vi "peak - geometry fit.vi"(10 "omega":dbl[](array[numeric]), 11 "linear z":cdb[](array[numeric])) -> (0 "gamma":dbl, 1 "omega":dbl)   [LabVIEW 2015]
uses:
  <vilib>/Analysis/6fits.llb/Curve Fitting Criteria.ctl
  <vilib>/Analysis/NI_AALPro.lvlib
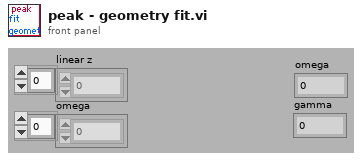
[diagram p1: front panel]
types:
  T1 = typedef "NI_AALPro.lvlib/Curve Fitting Criteria.ctl" = u16
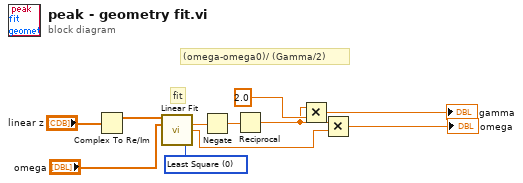
[diagram p0: block diagram]
diagram:
  w11 = T1 0 items=["Least Square", "Least Absolute Residual", "Bisquare"] ("method")
  # "(omega-omega0)/ (Gamma/2)"
  # "fit"
  n1 = Complex To Re/Im(x + iy="linear z") -> (x=w2:dbl[])  [unwired: 1 out]
  n2 = call <vilib>:"Linear Fit.vi"("Y"=w2, "X"="omega", "method"=w11) -> ("slope"=w9:dbl, "intercept"=w7:dbl)  [unwired: 8 in, 3 out]
  n3 = Negate(x=w9) -> (-x=w8:dbl)
  n4 = Reciprocal(x=w8) -> (1/x=w6:dbl)
  n5 = Multiply(x=w6, y=2.0) -> (x*y=→"gamma":dbl)
  n6 = Multiply(x=w6, y=w7) -> (x*y=→"omega":dbl)
